vi "InitFromString.vi"(9 "ActionStack String":string) -> (1 "ActionStack out":refnum<class "Stack.lvclass">)   [LabVIEW 2024, in "ActionStack.lvlib" / "Stack.lvclass"]
doc: "Splits string via /n (new line)\nThen check for Args which can be passed in the JKI SM style (action >> arg)\nCan be followed by // for comments\nArgument encoding (case insensitive):\n<B>Bools</B>\nT/True\nF/False\n<B>Numerics</B>\nu8.. u64: numeric value\ni8.. i64: signed numeric value\ns.. d: floating point value\n<B>Special Strings</B>\nPath: File/Folder Path\n<B>Default</B>\nstring"
uses:
  Stack.lvclass
  <vilib>/Utility/error.llb/Trim Whitespace One-Sided.vi
  Action/SingleWithPayload.vi
  Action/Action.lvclass
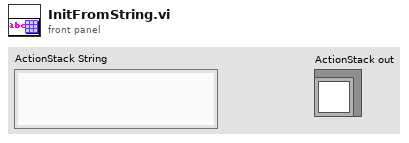
[diagram p1: front panel]
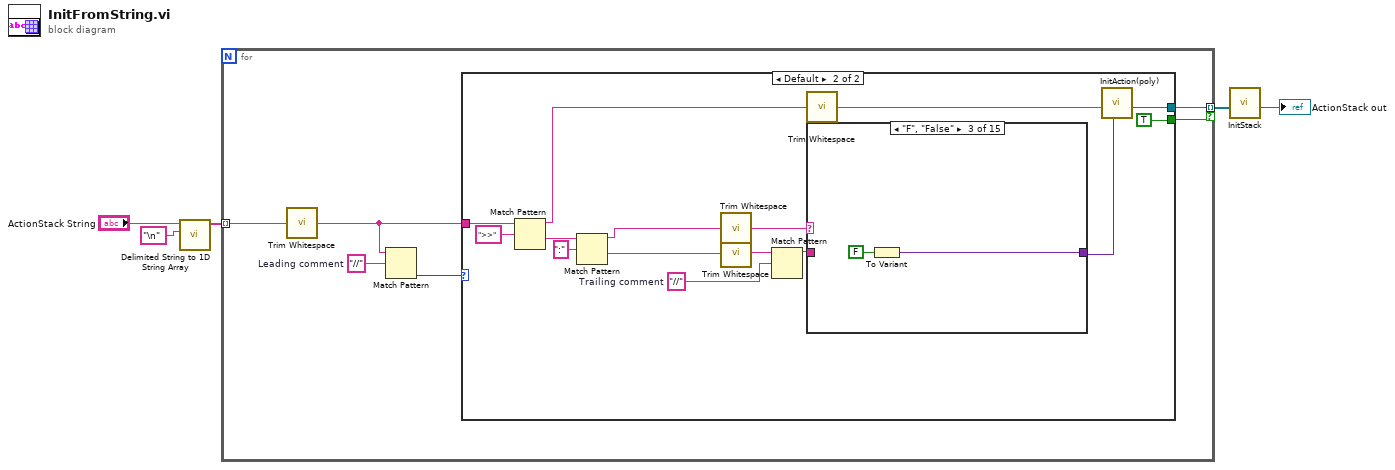
[diagram p0: block diagram]
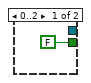
[diagram p2: hidden frame]
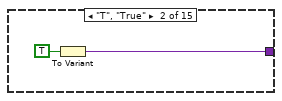
[diagram p4: hidden frame]
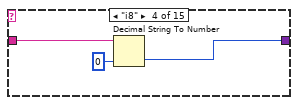
[diagram p5: hidden frame]
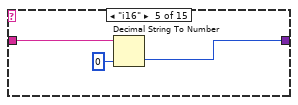
[diagram p6: hidden frame]
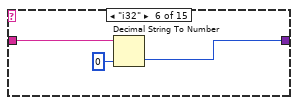
[diagram p7: hidden frame]
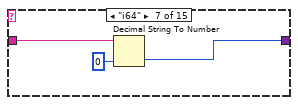
[diagram p8: hidden frame]
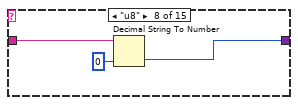
[diagram p9: hidden frame]
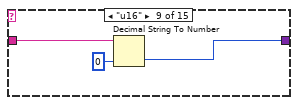
[diagram p10: hidden frame]
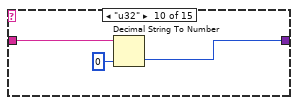
[diagram p11: hidden frame]
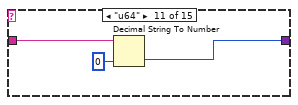
[diagram p12: hidden frame]
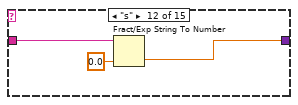
[diagram p13: hidden frame]
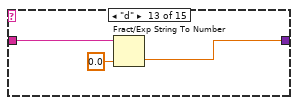
[diagram p14: hidden frame]
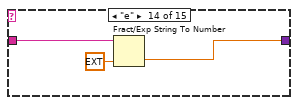
[diagram p15: hidden frame]
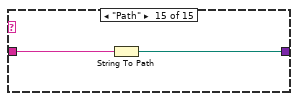
[diagram p16: hidden frame]
diagram:
  n1 = call <vilib>:"Delimited String to 1D String Array.vi"("delimiter"="\n", "delimited string"="ActionStack String") -> ("string array"=w3:string[])  [unwired: 9 in]
  n2 = for {
    tunnel: w3 -> [w9] mode=indexing
    tunnel: [w11] -> w2 mode=indexing if=w6
    w10 = "//"  # Leading comment
    n3 = call <vilib>:"Trim Whitespace.vi"("string"=w9) -> ("trimmed string"=w8:string)  [unwired: 1 in]
    n4 = Match Pattern(string=w8, regular expression=w10) -> (offset past match=w7:i32)  [unwired: 1 in, 3 out]
    n5 = case shown="Default" w7 {
      tunnel: [_ w14] -> w11
      tunnel: w8 -> [_ w17]
      tunnel: [FALSE TRUE] -> w6
      frame 0..2 {
      }
      frame Default {
        w18 = "//"  # Trailing comment
        n6 = Match Pattern(string=w17, regular expression=">>") -> (before substring=w26:string, after substring=w24:string)  [unwired: 1 in, 2 out]
        n7 = Match Pattern(string=w24, regular expression=":" ("search string/char (-)")) -> (before substring=w23:string, after substring=w22:string)  [unwired: 1 in, 2 out]
        n8 = call <vilib>:"Trim Whitespace.vi"("string"=w23) -> ("trimmed string"=w25:string)  [unwired: 1 in]
        n9 = call <vilib>:"Trim Whitespace.vi"("string"=w22) -> ("trimmed string"=w20:string)  [unwired: 1 in]
        n10 = Match Pattern(string=w20, regular expression=w18) -> (before substring=w19:string)  [unwired: 1 in, 3 out]
        n11 = call <vilib>:"Trim Whitespace.vi"("string"=w26) -> ("trimmed string"=w15:string)  [unwired: 1 in]
        n12 = case shown="\"F\", \"False\"" w25 {
          selector: w25 -> [w28 _ _ _ _ _ _ _ _ _ _ _ _ _ _]
          tunnel: [w28 w29 w31 w33 w36 w39 w42 w45 w48 w51 w54 w57 w60 w63 w66] -> w13
          tunnel: w19 -> [_ _ _ w35 w38 w41 w44 w47 w50 w53 w56 w59 w62 w65 w67]
          frame Default {
          }
          frame "T", "True" {
            n13 = To Variant(anything=TRUE) -> (Variant=w29:variant)
          }
          frame "F", "False" {
            n14 = To Variant(anything=FALSE) -> (Variant=w31:variant)
          }
          frame "i8" {
            n15 = Decimal String To Number(string=w35, default (0L)=i8 0 ("default (0 I32)")) -> (number=w33:i8)  [unwired: 1 in, 1 out]
          }
          frame "i16" {
            n16 = Decimal String To Number(string=w38, default (0L)=i16 0 ("default (0 I32)")) -> (number=w36:i16)  [unwired: 1 in, 1 out]
          }
          frame "i32" {
            n17 = Decimal String To Number(string=w41, default (0L)=0 ("default (0 I32)")) -> (number=w39:i32)  [unwired: 1 in, 1 out]
          }
          frame "i64" {
            n18 = Decimal String To Number(string=w44, default (0L)=i64 0 ("default (0 I32)")) -> (number=w42:i64)  [unwired: 1 in, 1 out]
          }
          frame "u8" {
            n19 = Decimal String To Number(string=w47, default (0L)=u8 0 ("default (0 I32)")) -> (number=w45:u8)  [unwired: 1 in, 1 out]
          }
          frame "u16" {
            n20 = Decimal String To Number(string=w50, default (0L)=u16 0 ("default (0 I32)")) -> (number=w48:u16)  [unwired: 1 in, 1 out]
          }
          frame "u32" {
            n21 = Decimal String To Number(string=w53, default (0L)=u32 0 ("default (0 I32)")) -> (number=w51:u32)  [unwired: 1 in, 1 out]
          }
          frame "u64" {
            n22 = Decimal String To Number(string=w56, default (0L)=u64 0 ("default (0 I32)")) -> (number=w54:u64)  [unwired: 1 in, 1 out]
          }
          frame "s" {
            n23 = Fract/Exp String To Number(string=w59, default (0 dbl)=sgl 0.0 ("default (0 I32)")) -> (number=w57:sgl)  [unwired: 2 in, 1 out]
          }
          frame "d" {
            n24 = Fract/Exp String To Number(string=w62, default (0 dbl)=0.0 ("default (0 I32)")) -> (number=w60:dbl)  [unwired: 2 in, 1 out]
          }
          frame "e" {
            n25 = Fract/Exp String To Number(string=w65, default (0 dbl)=ext 0.0 ("default (0 I32)")) -> (number=w63:ext)  [unwired: 2 in, 1 out]
          }
          frame "Path" {
            n26 = String To Path(string=w67) -> (path=w66:path)
          }
        }
        n27 = call-poly "InitAction(poly).vi"("Payload"=w13, "Action"=w15) -> ("ActionStack out"=w14:refnum<class "Action.lvclass">)  [unwired: 9 in]
      }
    }
  }
  n28 = call "InitStack.vi"("Action Stack"=w2) -> ("Stack"=→"ActionStack out":refnum<class "Stack.lvclass">)  [unwired: 10 in]
